vi "ActionVIOnLoad.vi"(8 "Error In":errorcluster, 11 "Device Item Ref In":T1 format="%.0x") -> (0 "Error Out":errorcluster, 3 "Device Item Ref out":T1 format="%.0x")   [LabVIEW 2018, in "NI-XNET Monitor System Explorer.lvlib"]
uses:
  NI-XNET Monitor System Explorer.lvlib
  <vilib>/NI Veristand/Custom Device API/Custom Device Item Ref.ctl
  <vilib>/NI VeriStand/Custom Device API/Custom Device API.lvlib
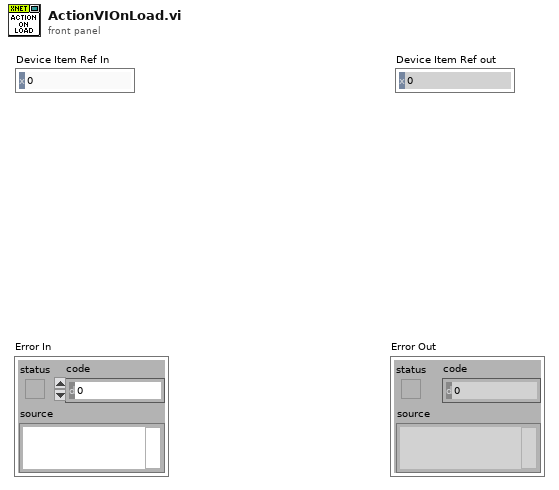
[diagram p1: front panel]
types:
  T1 = typedef "Custom Device API.lvlib/Custom Device Item Ref.ctl" = u64
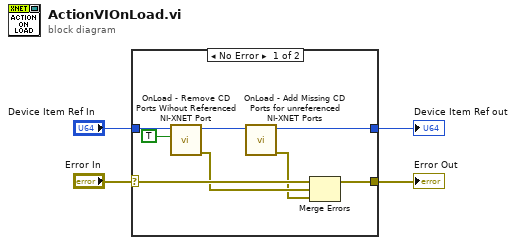
[diagram p0: block diagram]
diagram:
  n1 = case shown="No Error" "Error In" {
    selector: "Error In" -> [w12 w14]
    tunnel: [w9 w14] -> w3
    tunnel: "Device Item Ref In" -> [w11 w13]
    tunnel: [w10 w13] -> w1
    frame No Error {
      n2 = call "OnLoad - Remove CD Ports Wihout Referenced NI-XNET Port.vi"("Force Delete (F)"=TRUE, "Device Item Ref in in"=w11) -> ("error out"=w8:errorcluster, "Device Item Ref out"=w7:T1)  [unwired: 8 in]
      n3 = call "OnLoad - Add Missing CD Ports for unreferenced NI-XNET Ports.vi"("Device Item Ref in in"=w7) -> ("error out"=w6:errorcluster, "Device Item Ref out"=w10:T1)  [unwired: 9 in]
      n4 = Merge Errors(w12, w8, w6) -> (w9:errorcluster)
    }
    frame Error {
    }
  }
  "Error Out" <- w3
  "Device Item Ref out" <- w1
